vi "Channel ID to Tree Items.vi"(8 "error in (no error)":errorcluster, 9 "Channel ID":string, 11 "Application Data in":T2) -> (0 "error out":errorcluster, 1 "Settings":T1, 2 "Item":T1, 3 "Application Data out":T2)   [LabVIEW 2017, in "DSF Core.lvlib"]
uses:
  DSF Core.lvlib
  Main VI/Application Data.ctl
  <vilib>/NI/Memory Manager/Classes/Pointer/Pointer.lvclass
  Classes/Framework/Framework.lvclass
  Buffer Reader/Buffer Data.ctl
  Classes/Buffer/Buffer.lvclass
  Classes/Transfer Group Status/Status.lvclass
  Typedefs/DSF Engine Framework Configuration.ctl
  Typedefs/DSF Engine Plugin Configuration.ctl
  Typedefs/DSF Timing Info.ctl
  Typedefs/DSF Engine Plugin Thread Configuration.ctl
  Typedefs/DSF Settings Info.ctl
  Typedefs/DSF Engine Transfer Group Configuration.ctl
  Typedefs/DSF Direction.ctl
  Typedefs/DSF Engine Transfer Configuration.ctl
  Typedefs/DSF Byte Order.ctl
  Typedefs/DSF Engine Channel Configuration.ctl
  Typedefs/DSF Data Type.ctl
  Typedefs/DSF Timeout Behavior.ctl
  Tree Item.ctl
  Tree Item Type.ctl
  Builds/Data Sharing Framework/Current/Core/DSF Core.lvlibp/DSF Configuration API/Public/Read Item/Read Plugin.vi
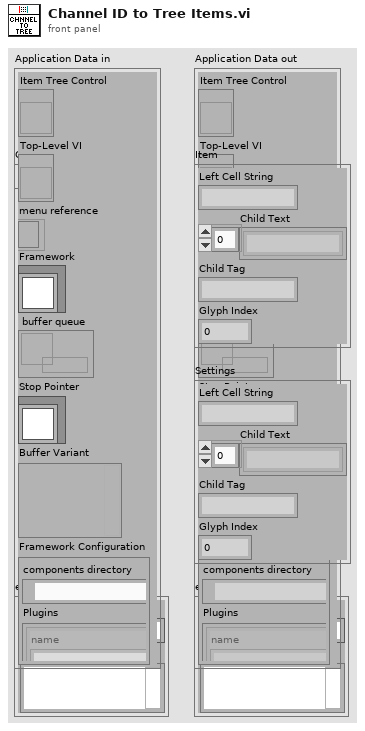
[diagram p1: front panel]
types:
  T1 = typedef "DSF Core.lvlib/Tree Item.ctl" = cluster{"Left Cell String":string, "Child Text":string[], "Child Tag":string, "Glyph Index":i32}
  T2 = typedef "DSF Core.lvlib/Application Data.ctl" = cluster{"Item Tree Control":refnum<vi>, "Top-Level VI":refnum<vi>, "menu reference":refnum<k9>, "Framework":refnum<class "Framework.lvclass">, "buffer queue":refnum<queue>, "Stop Pointer":refnum<class "Pointer.lvclass">, "Buffer Variant":variant, "Framework Configuration":T3}
  T3 = typedef "DSF Core.lvlib/DSF Engine Framework Configuration.ctl" = cluster{"components directory":path, "Plugins":T4[]}
  T4 = typedef "DSF Core.lvlib/DSF Engine Plugin Configuration.ctl" = cluster{"name":string, "components":string[], "cycle timing":T5, "threads":T6[], "Transfer Groups":T8[], "settings":T7}
  T5 = typedef "DSF Core.lvlib/DSF Timing Info.ctl" = cluster{"priority":u64, "decimation":u64, "offset":u64}
  T6 = typedef "DSF Core.lvlib/DSF Engine Plugin Thread Configuration.ctl" = cluster{"buffer converter settings":T7, "transceiver settings":T7, "processor":i32, "priority offset":i16}
  T7 = typedef "DSF Core.lvlib/DSF Settings Info.ctl" = cluster{"key":string, "value":string}[]
  T8 = typedef "DSF Core.lvlib/DSF Engine Transfer Group Configuration.ctl" = cluster{"name":string, "direction":T9, "cycle timing":T5, "thread index":i32, "settings":T7, "Transfers":T10[], "timeout behavior":T14}
  T9 = typedef "DSF Core.lvlib/DSF Direction.ctl" = enum8{"Tx", "Rx"}
  T10 = typedef "DSF Core.lvlib/DSF Engine Transfer Configuration.ctl" = cluster{"name":string, "byte order":T11, "settings":T7, "channels":T12[]}
  T11 = typedef "DSF Core.lvlib/DSF Byte Order.ctl" = enum8{"big-endian", "little-endian"}
  T12 = typedef "DSF Core.lvlib/DSF Engine Channel Configuration.ctl" = cluster{"string offset":u64, "string data type":T13, "engine data type":T13, "name":string, "settings":T7}
  T13 = typedef "DSF Core.lvlib/DSF Data Type.ctl" = enum8{"Bool", "SGL", "DBL", "I8", "I16", "I32", "I64", "U8", "U16", "U32", "U64"}
  T14 = typedef "DSF Core.lvlib/DSF Timeout Behavior.ctl" = enum8{"Increment Late Count", "Throw Error"}
  T15 = typedef "DSF Core.lvlib/Tree Item Type.ctl" = enum16{"Framework", "Plugin Group", "Plugin", "Group", "Transfer", "Buffer", "Channel"}
  T16 = typedef "DSF Core.lvlibp/DSF Plugin Info.ctl" = cluster{"components":string[], "timing":T17, "group ids":string[], "settings id":string, "threads":T18[]}
  T17 = typedef "DSF Core.lvlibp/DSF Timing Info.ctl" = cluster{"priority":u64, "decimation":u64, "offset":u64}
  T18 = typedef "DSF Core.lvlibp/DSF Engine Plugin Thread Configuration.ctl" = cluster{"buffer converter settings":T19, "transceiver settings":T19, "processor":i32, "priority offset":i16}
  T19 = typedef "DSF Core.lvlibp/DSF Settings Info.ctl" = cluster{"key":string, "value":string}[]
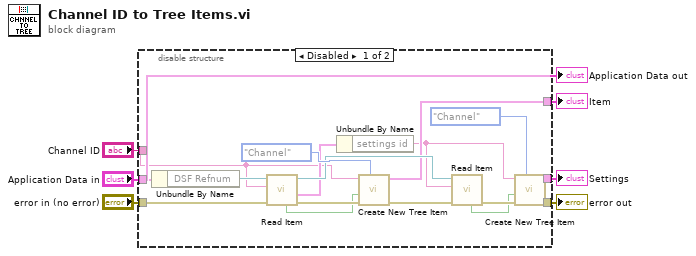
[diagram p0: block diagram]
diagram:
  n1 = disable-structure shown="Disabled" {
    disable-tunnel: [w21 _] -> w6
    disable-tunnel: "error in (no error)" -> [w17 _]
    disable-tunnel: "Application Data in" -> [w13 _]
    disable-tunnel: [w12 _] -> w3
    disable-tunnel: [w11 _] -> w2
    disable-tunnel: "Channel ID" -> [w10 _]
    frame Disabled {
      n2 = Unbundle By Name(w13) -> ("DSF Refnum"=w14:refnum<class "Configuration Session.lvclass">)
      n3 = call-poly "Read Item.vi"("error in (no error)"=w17, "Plugin ID"=w10, "Configuration Session in"=w14) -> ("error out"=w18:errorcluster, "value"=w15:T16, "Configuration Session out"=w16:refnum<class "Configuration Session.lvclass">, "found?"=w9:bool)  [unwired: 5 in]
      n4 = Unbundle By Name(w15) -> ("settings id"=w8:string)
      n5 = call "Create New Tree Item.vi"("Item Type"=Tree_Item_Type."Channel", "error in"=w18, "found?"=w9, "Left Cell String"=w10) -> ("error out"=w19:errorcluster, "Item"=w12:T1)  [unwired: 6 in]
      n6 = call-poly "Read Item.vi"("error in (no error)"=w19, "Plugin ID"=w8, "Configuration Session in"=w16) -> ("error out"=w20:errorcluster, "found?"=w7:bool)  [unwired: 5 in, 2 out]
      n7 = call "Create New Tree Item.vi"("Item Type"=Tree_Item_Type."Channel", "error in"=w20, "found?"=w7, "Left Cell String"=w8) -> ("error out"=w21:errorcluster, "Item"=w11:T1)  [unwired: 6 in]
    }
    frame Enabled {
    }
  }
  "error out" <- w6
  "Item" <- w3
  "Settings" <- w2
  "Application Data out" <- "Application Data in"
